vi "DrawClock.vi"(0 "Frame idx":i32=15, 5 "Draw Area Size":cluster{"Width":u32, "Height":u32}) -> (6 "Picture Draw Area Size":cluster{"Width":u32, "Height":u32}, 8 "clock picture":picture, 15 "Picture Rect":T1)   [LabVIEW 2024]
panel:
  in  "Case Constant\n(See Context Help) 2":bool=TRUE
  in  "Case Constant\n(See Context Help)":bool=TRUE
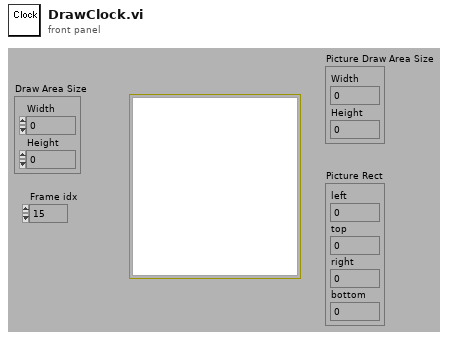
[diagram p1: front panel]
types:
  T1 = cluster{"left":i16, "top":i16, "right":i16, "bottom":i16}
  T2 = enum16{"User-specified Font", "Application Font", "System Font", "Dialog Font"}
  T3 = cluster{"Font Name:":string, "Size":i16, "Strikeout?":bool, "Italic?":bool, "Underline?":bool, "Outline?":bool, "Shadow?":bool, "Bold?":bool}
  T4 = cluster{"second":i32, "minute":i32, "hour":i32, "day of month":i32, "month":i32, "year":i32, "day of week":i32, "day of year":i32, "is DST":i32}
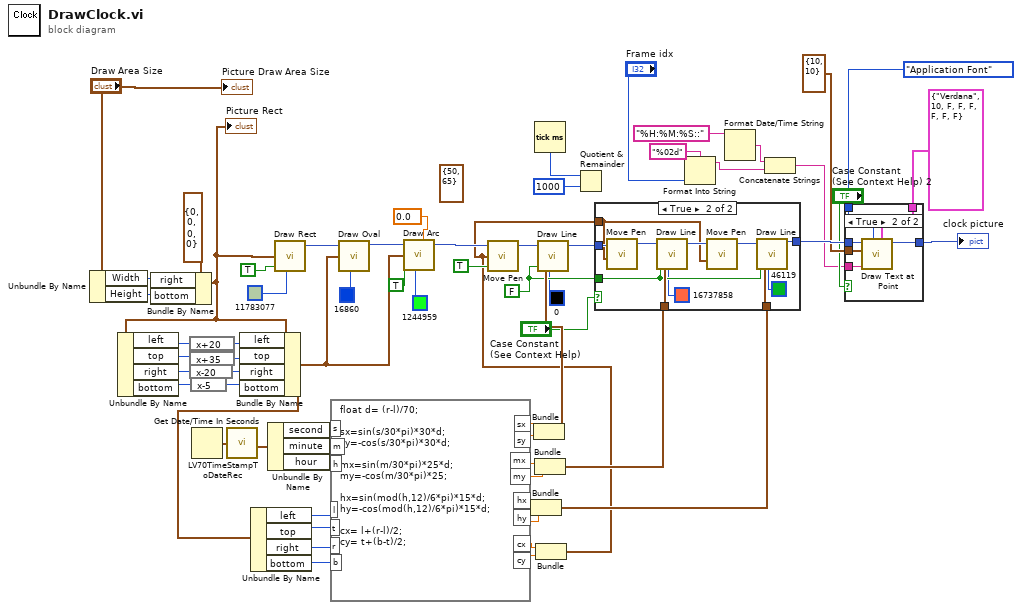
[diagram p0: block diagram]
diagram:
  w45 = FALSE ("absolute coordinates?(T)")
  (unwired) cluster{"x":i16, "y":i16} {"x"=50, "y"=65} ("new position")
  n1 = Unbundle By Name("Draw Area Size") -> ("Width"=w5:u32, "Height"=w4:u32)
  n2 = Bundle By Name(cluster=T1 {"left"=0, "top"=0, "right"=0, "bottom"=0} ("rect"), "right"=w5, "bottom"=w4) -> (w2:T1)
  "Picture Rect" <- w2
  n3 = Unbundle By Name(w2) -> ("left"=w21:i16, "top"=w14:i16, "right"=w15:i16, "bottom"=w16:i16)
  n4 = expression code="x+20"(w21) -> (w20:i16)
  n5 = expression code="x+35"(w14) -> (w19:i16)
  n6 = expression code="x-20"(w15) -> (w18:i16)
  n7 = expression code="x-5"(w16) -> (w17:i16)
  n8 = Get Date/Time In Seconds() -> (seconds since 1Jan1904=w1:timestamp)
  n9 = call <vilib>:"LV70TimeStampToDateRec.vi"("time stamp"=w1) -> ("date time rec"=w60:T4)
  n10 = Bundle By Name(cluster=w2, "left"=w20, "top"=w19, "right"=w18, "bottom"=w17) -> (w23:T1)
  n11 = Unbundle By Name(w23) -> ("left"=w13:i16, "top"=w12:i16, "right"=w11:i16, "bottom"=w10:i16)
  n12 = Unbundle By Name(w60) -> ("second"=w32:i32, "minute"=w57:i32, "hour"=w56:i32)
  n13 = call <vilib>:"Draw Rect.vi"("rect"=w2, "fill?(F)"=TRUE, "color(black)"=u32 11783077) -> ("new picture"=w64:picture)  [unwired: 2 in, 4 out]
  n14 = formula code="float d= (r-l)/70;\n\nsx=sin(s/30*pi)*30*d;\nsy=-cos(s/30*pi)*30*d;\n\nmx=sin(m/30*pi)*25*d;\nmy=-cos(m/30*pi)*25;\n\nhx=sin(mod(h,12)/6*pi)*15*d;\nhy=-cos(mod(h,12)/6*pi)*15*d;\n\ncx= l+(r-l)/2;\ncy= t+(b-t)/2;"("s"=w32, "m"=w57, "h"=w56, "l"=w13, "t"=w12, "r"=w11, "b"=w10) -> ("sx"=w55:dbl, "sy"=w54:dbl, "mx"=w51:dbl, "my"=w48:dbl, "hx"=w49:dbl, "hy"=w50:dbl, "cx"=w9:dbl, "cy"=w8:dbl)
  n15 = call <vilib>:"Draw Oval.vi"("picture"=w64, "rect"=w23, "color(black)"=u32 16860) -> ("new picture"=w38:picture)  [unwired: 2 in, 4 out]
  n16 = call <vilib>:"Draw Arc.vi"("picture"=w38, "rect"=w23, "fill?(F)"=TRUE, "color(black)"=u32 1244959, "arc size[degrees]"=0.0 ("y")) -> ("new picture"=w39:picture)  [unwired: 2 in, 2 out]
  n17 = Bundle("hx"=w49, "hy"=w50) -> (w46:cluster{"hx":dbl, "hy":dbl})  [unwired: 1 out]
  n18 = Bundle("sx"=w55, "sy"=w54) -> (w53:cluster{"sx":dbl, "sy":dbl})  [unwired: 1 out]
  n19 = Tick Count (ms)() -> (millisecond timer value=w27:u32)
  n20 = Bundle("mx"=w51, "my"=w48) -> (w47:cluster{"mx":dbl, "my":dbl})  [unwired: 1 out]
  n21 = Bundle("cx"=w9, "cy"=w8) -> (w7:cluster{"cx":dbl, "cy":dbl})  [unwired: 1 out]
  n22 = call <vilib>:"Move Pen.vi"("absolute coordinates?(T)"=TRUE, "new position"=w7, "picture"=w39) -> ("new picture"=w59:picture)  [unwired: 2 out]
  n23 = call <vilib>:"Draw Line.vi"("picture"=w59, "end point"=w53, "absolute coordinates?(T)"=w45, "color(black)"=u32 0) -> ("new picture"=w58:picture)  [unwired: 1 in, 4 out]
  n24 = Quotient & Remainder(x=w27, y=u32 1000) -> ()  [unwired: 2 out]
  n25 = case shown="True" "Case Constant\n(See Context Help)" {
    tunnel: w58 -> [w65 w76]
    tunnel: w7 -> [_ w72]
    tunnel: w47 -> [_ w71]
    tunnel: w46 -> [_ w70]
    tunnel: w45 -> [_ w69]
    tunnel: [w65 w66] -> w44
    frame False {
    }
    frame True {
      n26 = call <vilib>:"Move Pen.vi"("new position"=w72, "picture"=w76) -> ("new picture"=w75:picture)  [unwired: 1 in, 2 out]
      n27 = call <vilib>:"Draw Line.vi"("picture"=w75, "end point"=w71, "absolute coordinates?(T)"=w69, "color(black)"=u32 16737858) -> ("new picture"=w74:picture)  [unwired: 1 in, 4 out]
      n28 = call <vilib>:"Move Pen.vi"("new position"=w72, "picture"=w74) -> ("new picture"=w73:picture)  [unwired: 1 in, 2 out]
      n29 = call <vilib>:"Draw Line.vi"("picture"=w73, "end point"=w70, "absolute coordinates?(T)"=w69, "color(black)"=u32 46119) -> ("new picture"=w66:picture)  [unwired: 1 in, 4 out]
    }
  }
  n30 = Format Into String(format string="%02d" ("Format String"), "Frame idx") -> (resulting string=w29:string)  [unwired: 2 in, 1 out]
  n31 = Format Date/Time String(time format string (%c)="%H:%M:%S::" ("Format String")) -> (date/time string=w31:string)  [unwired: 2 out]
  n32 = Concatenate Strings(w31, w29) -> (w30:string)
  n33 = case shown="True" "Case Constant\n(See Context Help) 2" {
    tunnel: w44 -> [w77 w83]
    tunnel: [w77 w82] -> w43
    tunnel: cluster{"x":i16, "y":i16} {"x"=10, "y"=10} ("origin") -> [_ w81]
    tunnel: T3 {"Font Name:"="Verdana", "Size"=10, "Strikeout?"=FALSE, "Italic?"=FALSE, "Underline?"=FALSE, "Outline?"=FALSE, "Shadow?"=FALSE, "Bold?"=FALSE} ("[user-specified font]") -> [_ w80]
    tunnel: T2."Application Font" ("desired font(Application)") -> [_ w79]
    tunnel: w30 -> [_ w78]
    frame False {
    }
    frame True {
      n34 = call <vilib>:"Draw Text at Point.vi"("[user-specified font]"=w80, "desired font(Application)"=w79, "text"=w78, "origin"=w81, "picture"=w83) -> ("new picture"=w82:picture)  [unwired: 4 in, 2 out]
    }
  }
  "clock picture" <- w43
  "Picture Draw Area Size" <- "Draw Area Size"
